vi "Teleop Hopper Control.vi"(9 "D-Pad":T1, 10 "Button Cluster":T2, 11 "Axes":T3) -> ()   [LabVIEW 2016]
uses:
  Common Code/Gamepads/Axes Cluster.ctl
  Common Code/Gamepads/Button Cluster.ctl
  Common Code/Gamepads/D-Pad.ctl
  Robot Global Data.vi
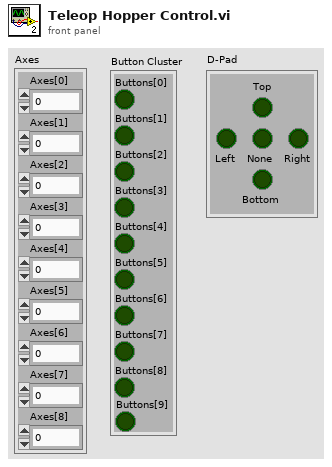
[diagram p1: front panel]
types:
  T1 = typedef "D-Pad.ctl" = cluster{"Top":bool, "Bottom":bool, "None":bool, "Right":bool, "Left":bool}
  T2 = typedef "Button Cluster.ctl" = cluster{"Buttons[0]":bool, "Buttons[1]":bool, "Buttons[2]":bool, "Buttons[3]":bool, "Buttons[4]":bool, "Buttons[5]":bool, "Buttons[6]":bool, "Buttons[7]":bool, "Buttons[8]":bool, "Buttons[9]":bool}
  T3 = typedef "Axes Cluster.ctl" = cluster{"Axes[0]":dbl, "Axes[1]":dbl, "Axes[2]":dbl, "Axes[3]":dbl, "Axes[4]":dbl, "Axes[5]":dbl, "Axes[6]":dbl, "Axes[7]":dbl, "Axes[8]":dbl}
  T4 = typedef "Hopper Command Cluster.ctl" = cluster{"Hopper Open?":bool}
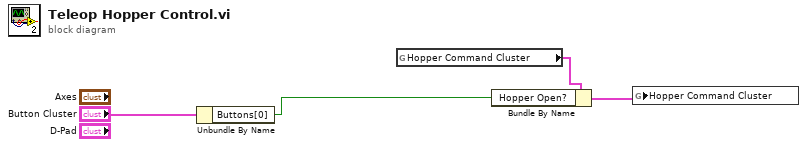
[diagram p0: block diagram]
diagram:
  n1 = Unbundle By Name("Button Cluster") -> ("Buttons[0]"=w1:bool)
  n2 = global read "Robot Global Data.vi" "Hopper Command Cluster"() -> (w3:T4)
  n3 = Bundle By Name(cluster=w3, "Hopper Open?"=w1) -> (w2:T4)
  n4 = global write "Robot Global Data.vi" "Hopper Command Cluster"(w2) -> ()
